vi "Read Base path.vi"(8 "error in (no error)":errorcluster, 11 "[Test Case] Build path in":refnum<class "[Test Case] Build path.lvclass">=refnum) -> (0 "error out":errorcluster, 2 "Base path":string, 3 "[Test Case] Build path out":refnum<class "[Test Case] Build path.lvclass">)   [LabVIEW 2016, in "Tests.lvlib" / "[Test Case] Build path.lvclass"]
uses:
  [Test Case] Build path.lvclass
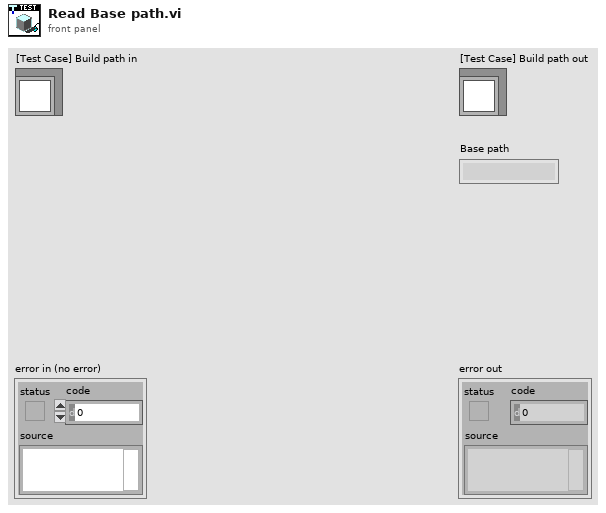
[diagram p1: front panel]
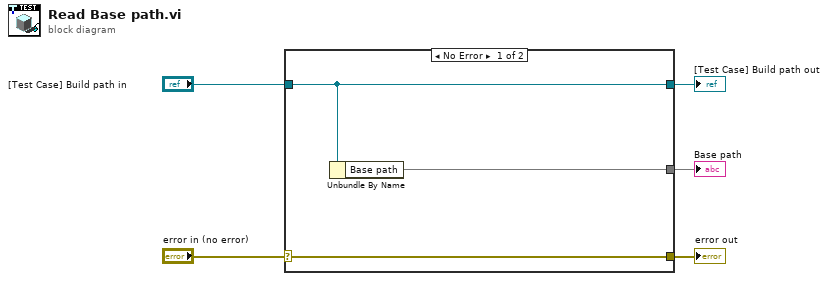
[diagram p0: block diagram]
diagram:
  n1 = case shown="No Error" "error in (no error)" {
    selector: "error in (no error)" -> [w8 w9]
    tunnel: [w8 w9] -> w4
    tunnel: [w7 w10] -> w2
    tunnel: "[Test Case] Build path in" -> [w7 w10]
    tunnel: [w6 _] -> w1
    frame No Error {
      n2 = Unbundle By Name(w7) -> ("Base path"=w6)
    }
    frame Error {
    }
  }
  "error out" <- w4
  "[Test Case] Build path out" <- w2
  "Base path" <- w1
